vi "Determine Module ID Index.vi"(8 "error in (no error)":errorcluster, 10 "Module ID":i32=-1, 11 "Select Module Ring Ref":refnum<vi>) -> (0 "error out":errorcluster, 2 "Module ID Index":i32)   [LabVIEW 2018, in "Timer Module.lvlib"]
uses:
  Timer Module.lvlib
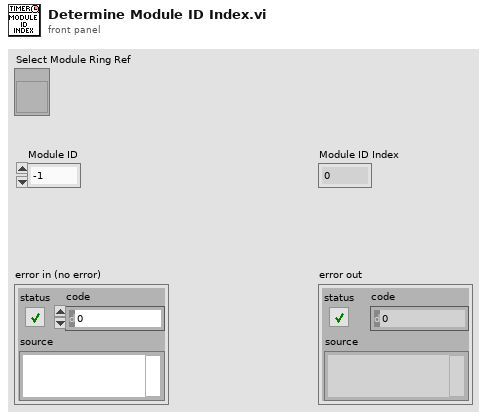
[diagram p1: front panel]
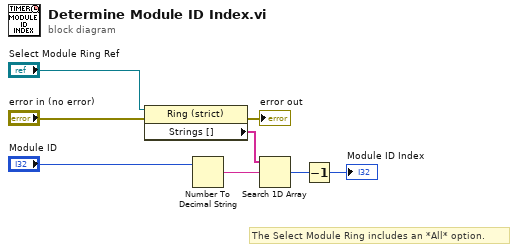
[diagram p0: block diagram]
diagram:
  # "The Select Module Ring includes an *All* option."
  n1 = property class="Ring (strict)"(reference="Select Module Ring Ref", error in="error in (no error)") -> (error out=→"error out":errorcluster, "Strings []"=w6:string[])  [unwired: 1 out]
  n2 = Number To Decimal String(number="Module ID") -> (decimal integer string=w5:string)  [unwired: 1 in]
  n3 = Search 1D Array(1D array=w6, element=w5) -> (index of element=w2:i32)  [unwired: 1 in]
  n4 = Decrement(x=w2) -> (x-1=→"Module ID Index":i32)
